vi "GT Get Crd Stop Dec.vi"(7 "pDecAbruptStop":dbl, 8 "error in (no error)":errorcluster caption="错误输入（无错误）", 9 "pDecSmoothStop":dbl, 10 "crd":i16, 11 "cardNum":i16) -> (0 "error out":errorcluster caption="错误输出", 1 "pDecSmoothStop out":dbl, 3 "function return":i16, 5 "pDecAbruptStop out":dbl)   [LabVIEW 2014, in "gts.lvlib"]
doc: "GT_API GT_GetCrdStopDec(short cardNum,short crd,double *pDecSmoothStop,double *pDecAbruptStop);"
uses:
  gts.lvlib
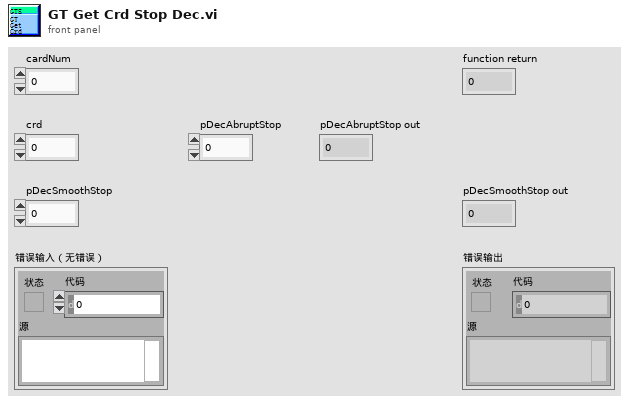
[diagram p1: front panel]
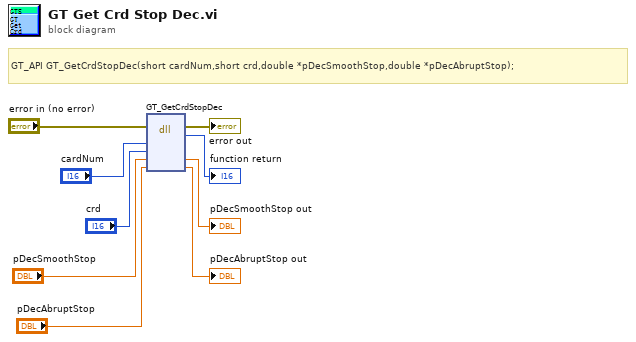
[diagram p0: block diagram]
diagram:
  # "GT_API GT_GetCrdStopDec(short cardNum,short crd,double *pDecSmoothStop,double *pDecAbruptStop);"
  n1 = dll-call lib="PTH2habs D固高科技资料GTS控制卡GTS卡18年上半年资料dllVC32bit\nmulti_cardgts.*" fn="GT_GetCrdStopDec"(error in="error in (no error)", "cardNum"="cardNum", "crd"="crd", "pDecSmoothStop"="pDecSmoothStop", "pDecAbruptStop"="pDecAbruptStop") -> (error out=→"error out":errorcluster, →"function return":i16, "pDecSmoothStop"=→"pDecSmoothStop out":dbl, "pDecAbruptStop"=→"pDecAbruptStop out":dbl)  [unwired: 4 in, 1 out]
